vi "GLOBAL_odour_protocol.vi"() -> ()   [LabVIEW 2016]
panel:
  in  "Protocol cluster":T1={"Sequence"=["SIMPLE 2A+", "SIMPLE 1A+"], "Rel. requency"=[1, 1], "Frequency"=[0.5, 0.5], "Sequence interval"=200.0, "Rarest sequence "=200.0, "Randomization"=2} {"Randomization" items=["None", "Simple shuffle", "Block"]}
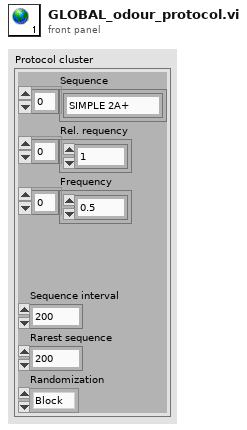
[diagram p1: front panel]
types:
  T1 = cluster{"Sequence":string[], "Rel. requency":u32[], "Frequency":dbl[], "Sequence interval":dbl, "Rarest sequence ":dbl, "Randomization":u16}
diagram:
